vi "DetectExtendCollision.vi"(4 "Ball":T1, 5 "Goal":dbl[](array[numeric]), 6 "Robot in":T2={"id"=0, "function"=enum."Attacker", "x"=0.0, "y"=0.0, "orientation"=0.0, "v_tangent"=0.0, "v_normal"=0.0, "v_ang"=0.0, "kick_x"=0.0, "kick_z"=0.0, "dribble"=FALSE, "Timestamp"=timestamp(0 s since 1904-01-01), "estimatives"={"est_v_tangent"=0.0, "est_v_normal"=0.0, "est_vx"=0.0, "est_vy"=0.0, "Pos Robot Est"=[]}, "dest_x_kick"=0.0, "dest_y_kick"=0.0, "Gap Coord"=[], "States"=enum."GoToTangent", "Path "=[], "Path  Smooth"=[], "Dest"=[], "vx_desired"=0.0, "vy_desired"=0.0, "slowBehavior"=FALSE, "VSSStates"=enum."Pass"}, 7 "Initial State":dbl[](array[numeric]), 8 "ignoreBall?":bool, 9 "enemy_robots":T2[](array[typedef]), 10 "Point":dbl[](array[numeric]), 11 "our_robots":T2[](array[typedef])) -> (2 "Collision":bool)   [LabVIEW 2023]
uses:
  Vision_class/Old vision/Controls/AI Robot.ctl
  Vision_class/Old vision/Controls/Functions Enum.ctl
  Vision_class/Old vision/Controls/AttackerStates.ctl
  Vision_class/Old vision/Controls/PathDests.ctl
  Vision_class/Old vision/Controls/PathDest.ctl
  Navigation/VSSNavigation/VSSAttackerStates.ctl
  Vision_class/Old vision/SSL Detection Frame Simple Estimator Cameras VelCmd Folder/Core/AI Ball.ctl
  Utilities_class/Utilities.lvclass
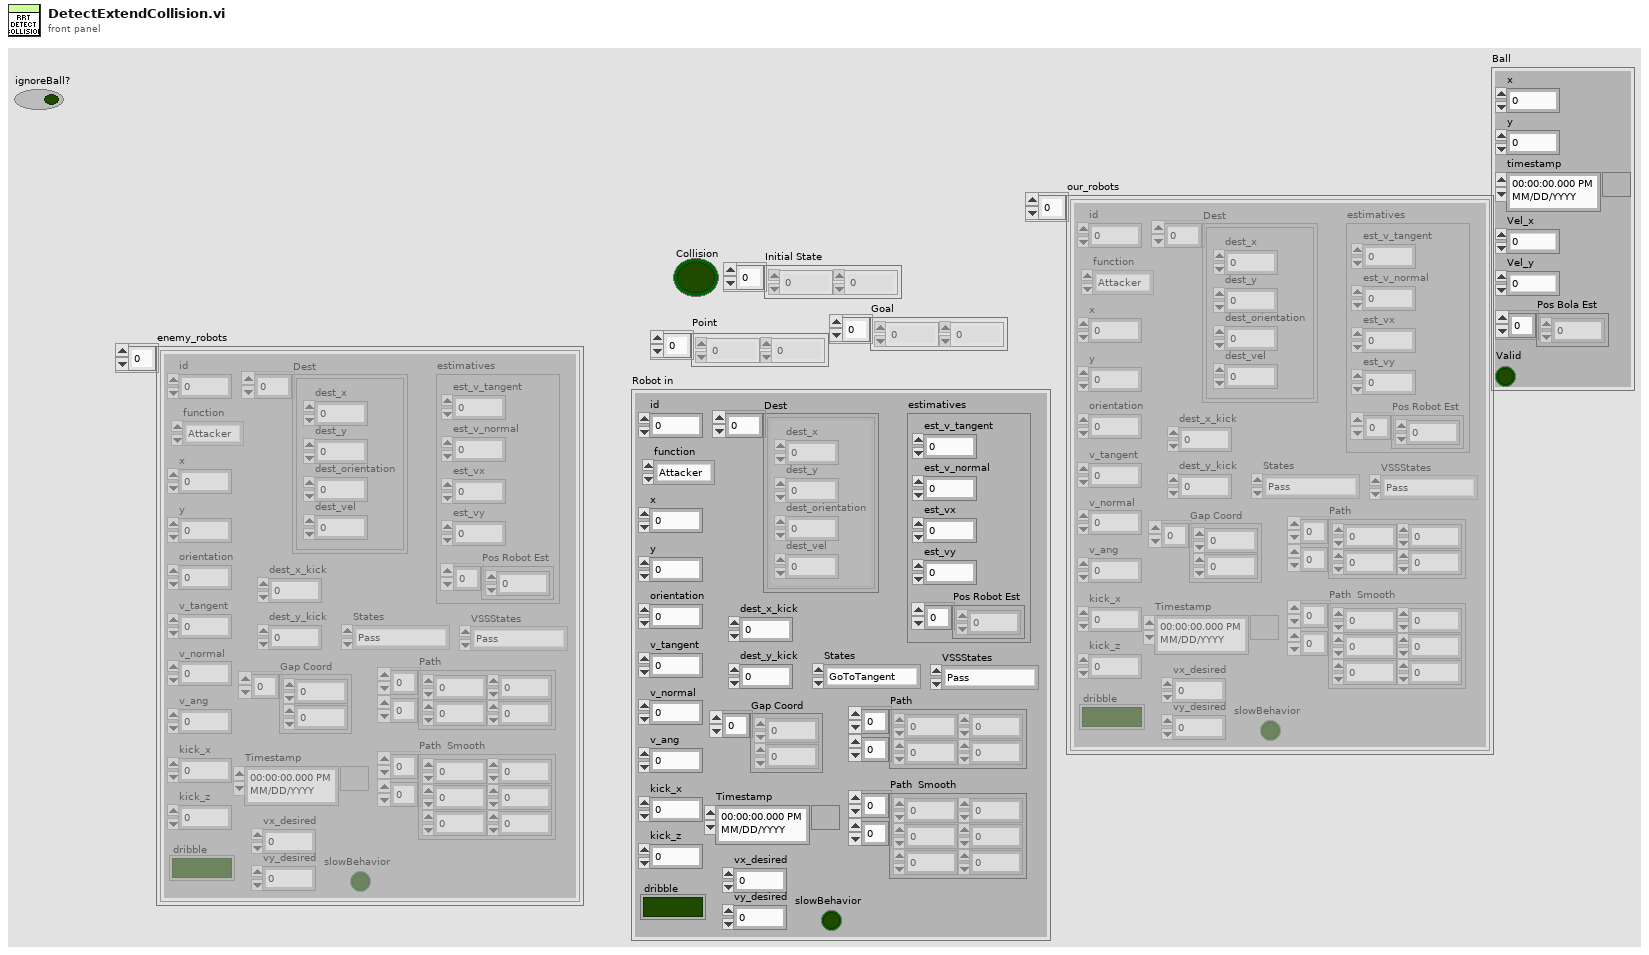
[diagram p1: front panel]
types:
  T1 = typedef "AI Ball.ctl" = cluster{"x":dbl, "y":dbl, "timestamp":timestamp, "Vel_x":dbl, "Vel_y":dbl, "Pos Bola Est":dbl[], "Valid":bool}
  T2 = typedef "AI Robot.ctl" = cluster{"id":u32, "function":T3, "x":dbl, "y":dbl, "orientation":dbl, "v_tangent":dbl, "v_normal":dbl, "v_ang":dbl, "kick_x":dbl, "kick_z":dbl, "dribble":bool, "Timestamp":timestamp, "estimatives":cluster{"est_v_tangent":dbl, "est_v_normal":dbl, "est_vx":dbl, "est_vy":dbl, "Pos Robot Est":dbl[]}, "dest_x_kick":dbl, "dest_y_kick":dbl, "Gap Coord":dbl[], "States":T4, "Path ":dbl[][], "Path  Smooth":dbl[][], "Dest":T5, "vx_desired":dbl, "vy_desired":dbl, "slowBehavior":bool, "VSSStates":T7}
  T3 = typedef "Functions Enum.ctl" = enum16{"2nd Striker", "Attacker", "Goalie", "Defender", "Striker", "Goto 0", "Dummy", "Kicker", "ZigZag 0", "ZigZag 1", "ZigZag 2", "ZigZag 3", "ZigZag 4", "ZigZag 5", "ZigZag 6", "ZigZag 7", "ZigZag 8", ""}
  T4 = typedef "AttackerStates.ctl" = enum16{"Pass", "GoToTangent", "BallGetting", "GoToKick", ""}
  T5 = typedef "PathDests.ctl" = T6[]
  T6 = typedef "PathDest.ctl" = cluster{"dest_x":dbl, "dest_y":dbl, "dest_orientation":dbl, "dest_vel":dbl}
  T7 = typedef "VSSAttackerStates.ctl" = enum16{"Pass", "GoToTangent", "BallGetting", "GoToKick", "Rotate anti-clockwise", "Rotate Clockwise", ""}
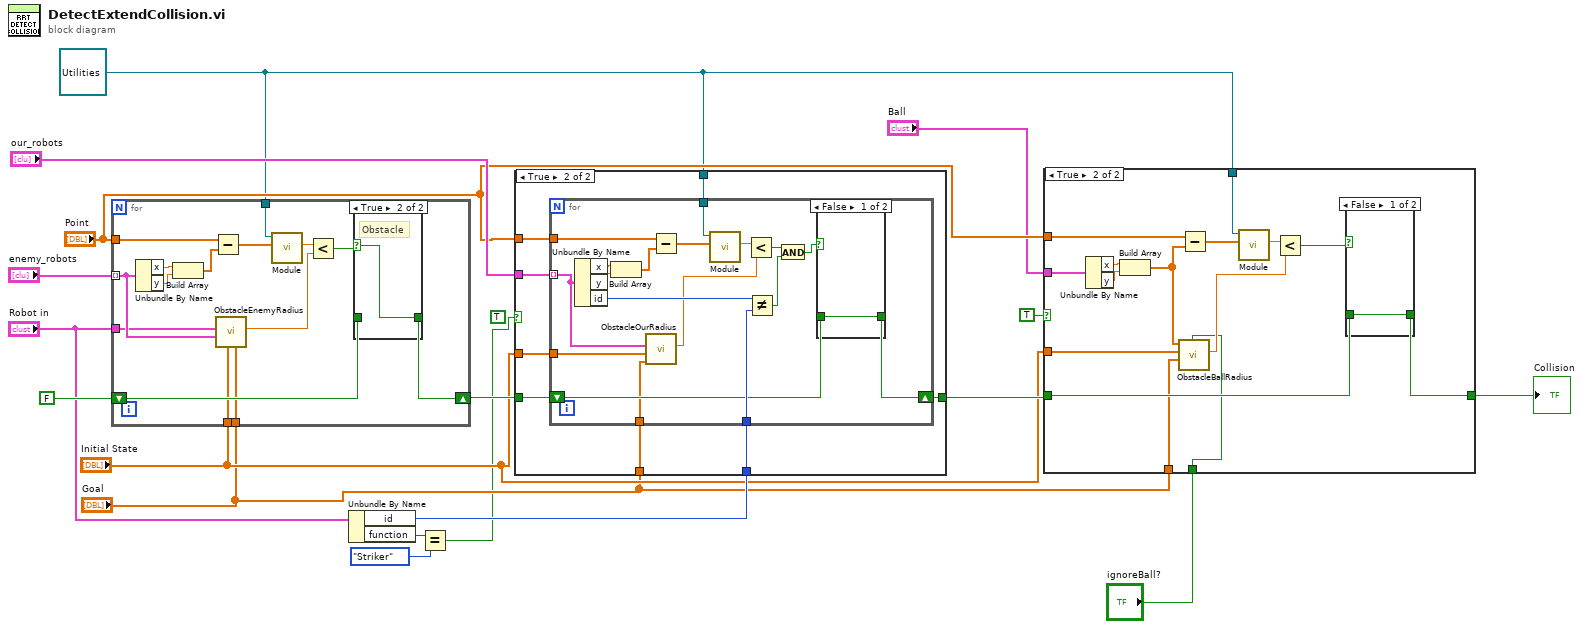
[diagram p0: block diagram]
diagram:
  w2 = refnum<class "Utilities.lvclass"> refnum ("Utilities in")
  (unwired) TRUE
  n1 = for {
    tunnel: "enemy_robots" -> [w23] mode=indexing
    tunnel: "Point" -> [w30]
    shift-right: [w25] -> w13
    shift-left: FALSE -> [w26]
    tunnel: "Robot in" -> [w22]
    tunnel: "Initial State" -> [w21]
    tunnel: "Goal" -> [w20]
    tunnel: w2 -> [w19]
    n2 = Unbundle By Name(w23) -> ("x"=w33:dbl, "y"=w32:dbl)
    n3 = Build Array(w33, w32) -> (w31:dbl[])
    n4 = Subtract(x=w30, y=w31) -> (x-y=w29:dbl[])
    n5 = call "ObstacleEnemyRadius.vi"("Goal"=w20, "Initial State"=w21, "Robot enemy"=w23, "Robot in"=w22) -> ("obstacle enemy radius"=w24:dbl)  [unwired: 7 in]
    n6 = call "Module.vi"("2D vector"=w29, "Utilities in"=w19) -> ("Modulo"=w28:dbl)  [unwired: 7 in, 2 out]
    n7 = Less?(x=w28, y=w24) -> (x < y?=w27:bool)
    n8 = case shown="True" w27 {
      selector: w27 -> [_ w35]
      tunnel: w26 -> [w34 _]
      tunnel: [w34 w35] -> w25
      frame False {
      }
      frame True {
        # "Obstacle"
      }
    }
  }
  n9 = Unbundle By Name("Robot in") -> ("id"=w14:u32, "function"=w5:T3)
  n10 = Equal?(x=w5, y=Functions_Enum."Striker") -> (x = y?=w3:bool)
  n11 = case shown="True" w3 {
    tunnel: w13 -> [w36 w44]
    tunnel: "our_robots" -> [_ w43]
    tunnel: "Point" -> [_ w42]
    tunnel: [w36 w41] -> w10
    tunnel: w14 -> [_ w40]
    tunnel: "Initial State" -> [_ w39]
    tunnel: "Goal" -> [_ w38]
    tunnel: w2 -> [_ w37]
    frame False {
    }
    frame True {
      n12 = for {
        tunnel: w43 -> [w46] mode=indexing
        tunnel: w42 -> [w59]
        shift-right: [w56] -> w41
        shift-left: w44 -> [w50]
        tunnel: w40 -> [w51]
        tunnel: w39 -> [w48]
        tunnel: w38 -> [w47]
        tunnel: w37 -> [w45]
        n13 = Unbundle By Name(w46) -> ("x"=w62:dbl, "y"=w61:dbl, "id"=w52:u32)
        n14 = Build Array(w62, w61) -> (w60:dbl[])
        n15 = call "ObstacleOurRadius.vi"("Goal"=w47, "Initial State"=w48, "other robot"=w46) -> ("obstacle enemy radius"=w49:dbl)  [unwired: 8 in]
        n16 = Subtract(x=w59, y=w60) -> (x-y=w58:dbl[])
        n17 = call "Module.vi"("2D vector"=w58, "Utilities in"=w45) -> ("Modulo"=w57:dbl)  [unwired: 7 in, 2 out]
        n18 = Less?(x=w57, y=w49) -> (x < y?=w55:bool)
        n19 = Not Equal?(x=w52, y=w51) -> (x != y?=w53:bool)
        n20 = And(x=w55, y=w53) -> (x .and. y?=w54:bool)
        n21 = case shown="False" w54 {
          selector: w54 -> [_ w64]
          tunnel: w50 -> [w63 _]
          tunnel: [w63 w64] -> w56
          frame False {
          }
          frame True {
            # "Obstacle"
          }
        }
      }
    }
  }
  n22 = case shown="True" TRUE {
    tunnel: w10 -> [w65 w80]
    tunnel: "Ball" -> [_ w79]
    tunnel: "Point" -> [_ w78]
    tunnel: [w65 w77] -> w12
    tunnel: "Initial State" -> [_ w70]
    tunnel: "Goal" -> [_ w69]
    tunnel: w2 -> [_ w67]
    tunnel: "ignoreBall?" -> [_ w66]
    frame False {
    }
    frame True {
      n23 = Unbundle By Name(w79) -> ("x"=w73:dbl, "y"=w72:dbl)
      n24 = Build Array(w73, w72) -> (w71:dbl[])
      n25 = call "ObstacleBallRadius.vi"("ignoreBall?"=w66, "Goal"=w69, "Initial State"=w70, "ball"=w71) -> ("obstacle enemy radius"=w68:dbl)  [unwired: 7 in]
      n26 = Subtract(x=w78, y=w71) -> (x-y=w76:dbl[])
      n27 = call "Module.vi"("2D vector"=w76, "Utilities in"=w67) -> ("Modulo"=w75:dbl)  [unwired: 7 in, 2 out]
      n28 = Less?(x=w75, y=w68) -> (x < y?=w74:bool)
      n29 = case shown="False" w74 {
        selector: w74 -> [_ w82]
        tunnel: w80 -> [w81 _]
        tunnel: [w81 w82] -> w77
        frame False {
        }
        frame True {
          # "Obstacle"
        }
      }
    }
  }
  "Collision" <- w12
